vi "Temp Fault Handler.vi"(6 "Fault Count In":u64, 9 "LAB deg C 2":T1, 10 "LAB deg C Prev":T1, 11 "Fault":bool) -> (0 "Fault Count Out":u64, 3 "LAB deg C Current":T1)   [LabVIEW 2017]
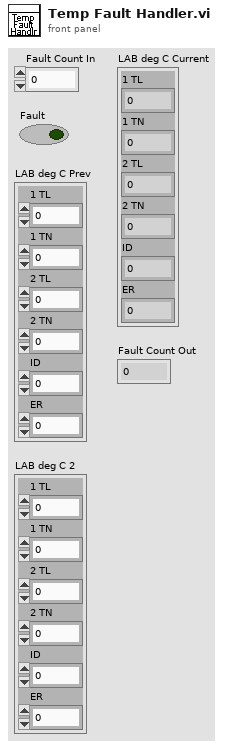
[diagram p1: front panel]
types:
  T1 = cluster{"1 TL":dbl, "1 TN":dbl, "2 TL":dbl, "2 TN":dbl, "ID":dbl, "ER":dbl}
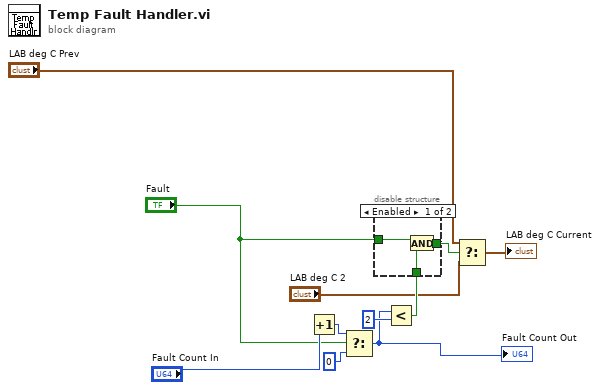
[diagram p0: block diagram]
diagram:
  n1 = Increment(x="Fault Count In") -> (x+1=w2:u64)
  n2 = Select(t=w2, s="Fault", f=u64 0) -> (s? t:f=w8:u64)
  "Fault Count Out" <- w8
  n3 = Less?(x=w8, y=u64 2) -> (x < y?=w11:bool)
  n4 = disable-structure shown="Enabled" {
    disable-tunnel: w11 -> [w14 _]
    disable-tunnel: [w13 _] -> w10
    disable-tunnel: "Fault" -> [w12 _]
    frame Enabled {
      n5 = And(x=w12, y=w14) -> (x .and. y?=w13:bool)
    }
    frame Disabled {
    }
  }
  n6 = Select(t="LAB deg C Prev", s=w10, f="LAB deg C 2") -> (s? t:f=→"LAB deg C Current":T1)
